vi "Metronome.vi"() -> ()   [LabVIEW 2014]
panel:
  in  "stop":bool
  in  "Beats Per Minute":dbl
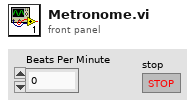
[diagram p1: front panel]
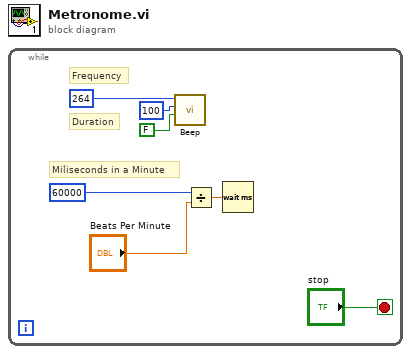
[diagram p0: block diagram]
diagram:
  n1 = while {
    stop <- "stop" stop-if-true
    # "Miliseconds in a Minute"
    # "Duration"
    # "Frequency"
    n2 = call <vilib>:"Beep.vi"("use system alert? (T)"=FALSE, "duration (msec)"=u32 100, "frequency (Hz)"=u32 264) -> ()  [unwired: 9 in]
    n3 = Divide(x=60000, y="Beats Per Minute") -> (x/y=w1:dbl)
    n4 = Wait (ms)(milliseconds to wait=w1) -> ()  [unwired: 1 out]
  }
